vi "电源设置.vi"(8 "error in (no error)":errorcluster caption="错误输入（无错误）", 10 "数值":dbl) -> (0 "error out":errorcluster caption="错误输出")   [LabVIEW 2012]
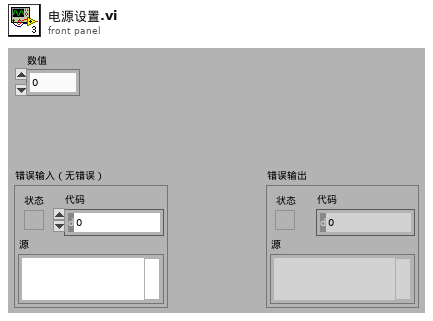
[diagram p1: front panel]
types:
  T1 = typedef "控件 3.ctl" = enum16{"初始化", "读取", "写入", "退出"}
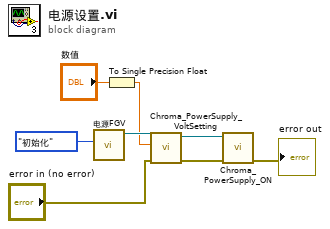
[diagram p0: block diagram]
diagram:
  n1 = call "电源FGV.vi"("枚举"=控件_3."初始化") -> ("VISA资源名称输出"=w7:refnum<visa-resource-name>)  [unwired: 9 in, 1 out]
  n2 = To Single Precision Float(number="数值") -> (single precision float=w1:sgl)
  n3 = call "Chroma_PowerSupply_VoltSetting.vi"("错误输入（无错误）"="error in (no error)", "VoltageSetting"=w1, "VISA资源名称"=w7) -> ("错误输出"=w4:errorcluster, "VISA资源名称输出"=w2:refnum<visa-resource-name>)  [unwired: 7 in]
  n4 = call "Chroma_PowerSupply_ON.vi"("错误输入（无错误）"=w4, "VISA资源名称"=w2) -> ("错误输出"=→"error out":errorcluster)  [unwired: 8 in, 1 out]
